vi "write path.vi"(8 "error in (no error)":errorcluster, 10 "Path Cluster":T2, 11 "CL57RS in":refnum<class "CL57RS.lvclass">) -> (0 "error out":errorcluster, 3 "CL57RS out":refnum<class "CL57RS.lvclass">)   [LabVIEW 2025, in "Motor.lvlib" / "CL57RS.lvclass"]
uses:
  CL57RS.lvclass
  Stepper/Path Mode.ctl
  CL57RS.lvclass/CL57RS.ctl
  Motor.lvlib
panel:
  out "appended array":u32[](array[numeric])
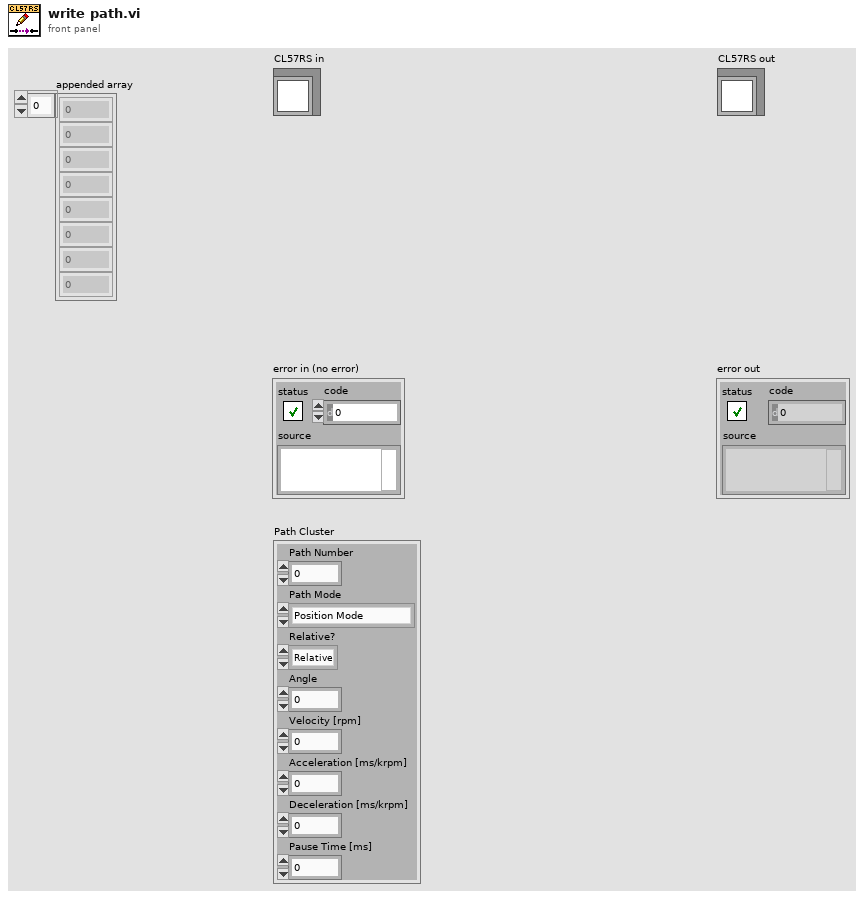
[diagram p1: front panel]
types:
  T1 = typedef "Motor.lvlib/Path Mode.ctl" = enum16{"Position Mode", "Velocity Mode", "Homing Mode"}
  T2 = cluster{"Path Number":i32, "Path Mode":T1, "Relative?":enum16{"Relative", "Absolute"}, "Angle":dbl, "Velocity [rpm]":i32, "Acceleration [ms/krpm]":i32, "Deceleration [ms/krpm]":i32, "Pause Time [ms]":i32}
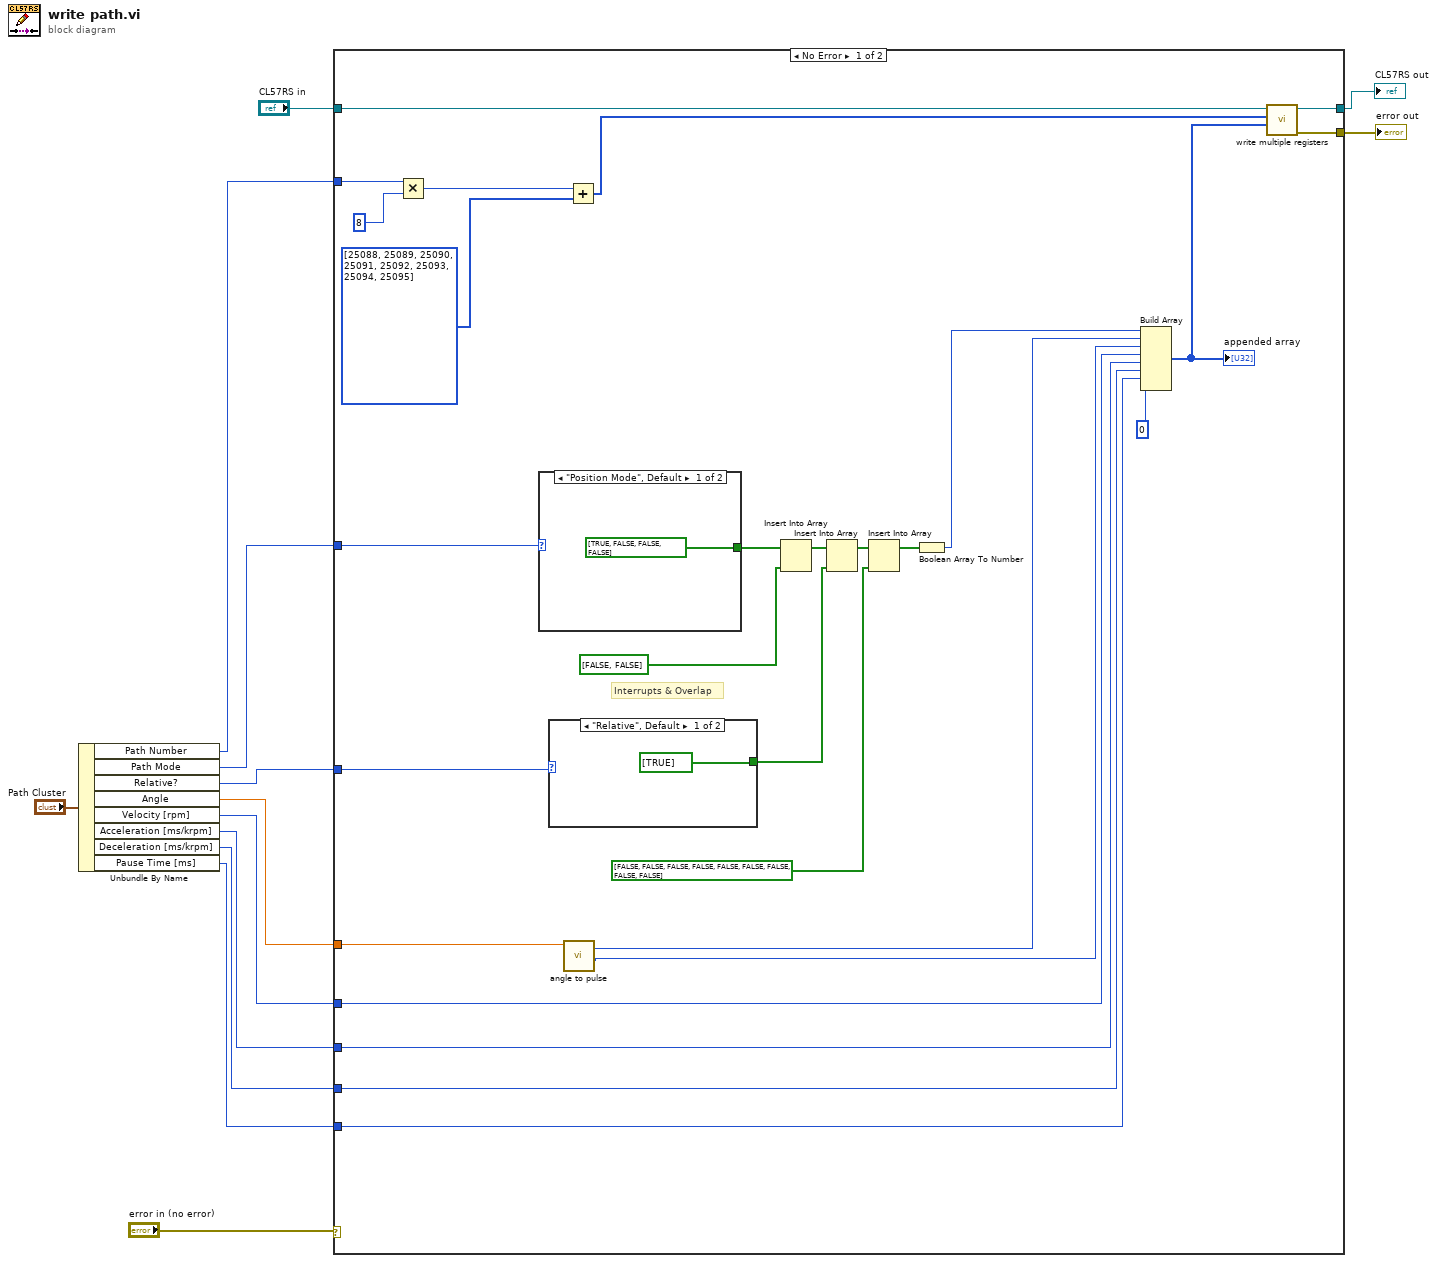
[diagram p0: block diagram]
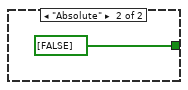
[diagram p2: hidden frame]
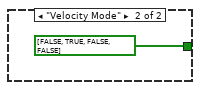
[diagram p3: hidden frame]
diagram:
  n1 = Unbundle By Name("Path Cluster") -> ("Path Number"=w12:i32, "Path Mode"=w11:T1, "Relative?"=w10:enum16{"Relative", "Absolute"}, "Angle"=w9:dbl, "Velocity [rpm]"=w8:i32, "Acceleration [ms/krpm]"=w7:i32, "Deceleration [ms/krpm]"=w6:i32, "Pause Time [ms]"=w5:i32)
  n2 = case shown="No Error" "error in (no error)" {
    selector: "error in (no error)" -> [_ w46]
    tunnel: [w17 w46] -> w2
    tunnel: [w39 w45] -> w3
    tunnel: "CL57RS in" -> [w40 w45]
    tunnel: w12 -> [w38 _]
    tunnel: w11 -> [w33 _]
    tunnel: w10 -> [w32 _]
    tunnel: w9 -> [w16 _]
    tunnel: w8 -> [w23 _]
    tunnel: w7 -> [w22 _]
    tunnel: w6 -> [w21 _]
    tunnel: w5 -> [w20 _]
    frame No Error {
      # "Interrupts & Overlap"
      n3 = Multiply(x=w38, y=8) -> (x*y=w36:i32)
      n4 = case shown="\"Position Mode\", Default" w33 {
        tunnel: [bool[] [TRUE, FALSE, FALSE, FALSE] bool[] [FALSE, TRUE, FALSE, FALSE]] -> w31
        frame "Position Mode", Default {
        }
        frame "Velocity Mode" {
        }
      }
      n5 = case shown="\"Relative\", Default" w32 {
        tunnel: [bool[] [TRUE] bool[] [FALSE]] -> w28
        frame "Relative", Default {
        }
        frame "Absolute" {
        }
      }
      n6 = call "angle to pulse.vi"("Angle"=w16) -> ("lo(x)"=w14:u16, "hi(x)"=w15:u16)  [unwired: 8 in, 1 out]
      n7 = Add(x=w36, y=u16[] [25088, 25089, 25090, 25091, 25092, 25093, 25094, 25095] ("addresses")) -> (x+y=w34:i32[])
      n8 = Insert Into Array(array=w31, new element=bool[] [FALSE, FALSE]) -> (w29:bool[])  [unwired: 1 in]
      n9 = Insert Into Array(array=w29, new element=w28) -> (w27:bool[])  [unwired: 1 in]
      n10 = Insert Into Array(array=w27, new element=bool[] [FALSE, FALSE, FALSE, FALSE, FALSE, FALSE, FALSE, FALSE, FALSE]) -> (w25:bool[])  [unwired: 1 in]
      n11 = Boolean Array To Number(Boolean array=w25) -> (number=w24:u32)
      n12 = Build Array(w24, w15, w14, w23, w22, w21, w20, u32 0 ("element")) -> (w18:u32[])
      "appended array" <- w18
      n13 = call "write multiple registers.vi"("register values"=w18, "addresses"=w34, "CL57RS in"=w40) -> ("error out"=w17:errorcluster, "CL57RS out"=w39:refnum<class "CL57RS.lvclass">)  [unwired: 7 in]
    }
    frame Error {
    }
  }
  "error out" <- w2
  "CL57RS out" <- w3
